vi "ZCAN_Transmit.vi"(0 "can_index_handle":u32, 1 "ID":u32 format="0x%08x", 2 "数据长度":u8 max=8, 3 "DATA":T1, 4 "每次发送帧数":u32=1, 5 "error in (no error)":errorcluster caption="错误输入（无错误）", 6 "帧类型":u32(ring) items=["标准帧", "扩展帧"], 8 "帧格式":u32(ring) items=["数据帧", "远程帧"], 10 "发送方式":u32(ring) items=["正常发送", "单次发送", "自发自收", "单次自发自收"]) -> (19 "error out":errorcluster caption="错误输出")   [LabVIEW 2018]
doc: "该函数用于发送CAN报文。"
uses:
  bin/zlgcan_wrap.dll
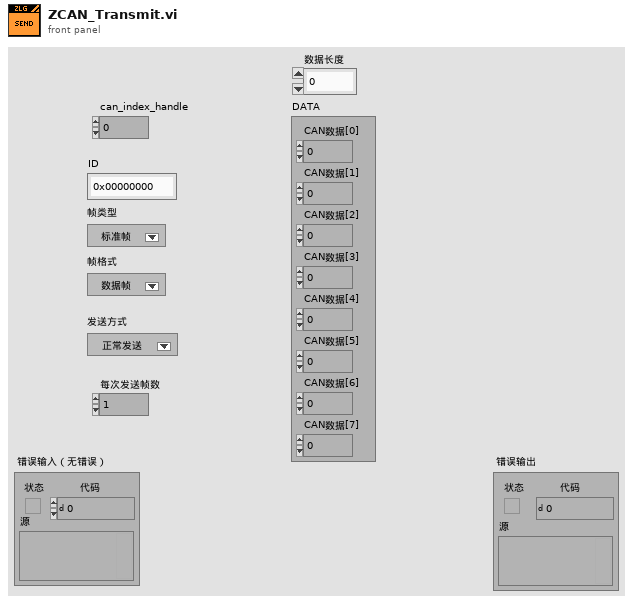
[diagram p1: front panel]
types:
  T1 = cluster{"CAN数据[0]":u8, "CAN数据[1]":u8, "CAN数据[2]":u8, "CAN数据[3]":u8, "CAN数据[4]":u8, "CAN数据[5]":u8, "CAN数据[6]":u8, "CAN数据[7]":u8}
  T2 = cluster{u32, "数据长度":u8, u8, u8, u8, "DATA":cluster{"CAN数据[0]":u8, "CAN数据[1]":u8, "CAN数据[2]":u8, "CAN数据[3]":u8, "CAN数据[4]":u8, "CAN数据[5]":u8, "CAN数据[6]":u8, "CAN数据[7]":u8}, "发送方式":u32}
  T3 = cluster{u32, "数据长度":u8, u8, u8, u8, "DATA":cluster{"CAN数据[0]":u8, "CAN数据[1]":u8, "CAN数据[2]":u8, "CAN数据[3]":u8, "CAN数据[4]":u8, "CAN数据[5]":u8, "CAN数据[6]":u8, "CAN数据[7]":u8}, "发送方式":u32}[]
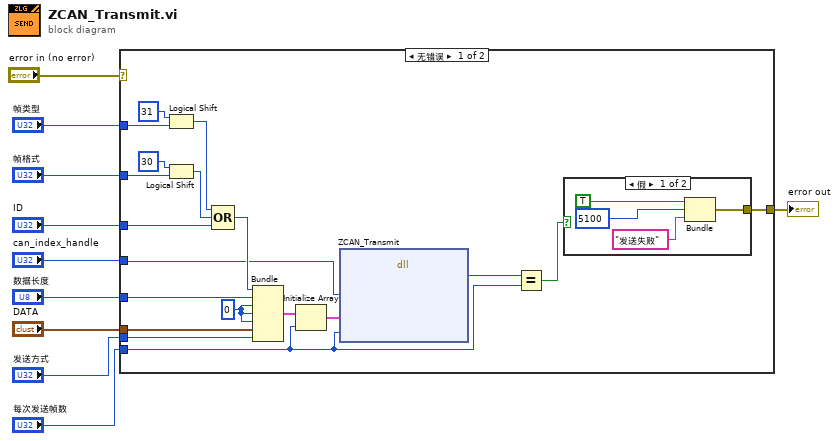
[diagram p0: block diagram]
diagram:
  n1 = case shown="无错误" "error in (no error)" {
    selector: "error in (no error)" -> [_ w34]
    tunnel: [w15 w34] -> w9
    tunnel: "ID" -> [w21 _]
    tunnel: "帧格式" -> [w20 _]
    tunnel: "帧类型" -> [w19 _]
    tunnel: "发送方式" -> [w18 _]
    tunnel: "数据长度" -> [w17 _]
    tunnel: "DATA" -> [w16 _]
    tunnel: "每次发送帧数" -> [w14 _]
    tunnel: "can_index_handle" -> [w11 _]
    frame No Error {
      w29 = u8 0
      n2 = Logical Shift(y=i16 31, x=w19) -> (x << y=w26:u32)
      n3 = Logical Shift(y=i16 30, x=w20) -> (x << y=w23:u32)
      n4 = Compound Arithmetic op=OR ("复合运算")(w26, w23, w21) -> (w22:u32)
      n5 = Bundle ("捆绑")(w22, "数据长度"=w17, w29, w29, w29, "DATA"=w16, "发送方式"=w18) -> (w28:T2)  [unwired: 1 in]
      n6 = Initialize Array(w28, w14) -> (w27:T3)
      n7 = dll-call lib="PTH2Fabs D\nUSBCANFD DEMO20200512USBCAN-I系列binzlgcan_wrap.dll" fn="ZCAN_Transmit"("通道句柄"=w11, "数据帧数组"=w27, "数据帧数"=w14) -> ("返回类型"=w13:u32)  [unwired: 6 in, 2 out]
      n8 = Equal?(x=w13, y=w14) -> (x = y?=w12:bool)
      n9 = case shown="假" w12 {
        tunnel: [w30 _] -> w15
        frame False {
          n10 = Bundle("status"=TRUE, "code"=5100, "消息"="发送失败") -> (w30:cluster{"status":bool, "code":i32, "消息":string})  [unwired: 1 in]
        }
        frame True {
        }
      }
    }
    frame Error {
    }
  }
  "error out" <- w9
